vi "Write then Read.vi"(8 "error in (no error)":errorcluster, 9 "milliseconds to wait":u32, 10 "Write":string, 11 "Serial in":refnum<class "Serial.lvclass">) -> (0 "error out":errorcluster, 2 "Read":string, 3 "Serial out":refnum<class "Serial.lvclass">)   [LabVIEW 2021, in "Serial.lvclass"]
uses:
  Serial.lvclass
  Serial.lvclass/Serial.ctl
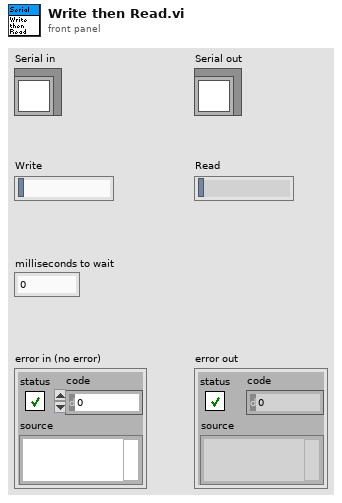
[diagram p1: front panel]
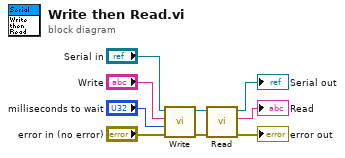
[diagram p0: block diagram]
diagram:
  n1 = call-dynamic "Write.vi"("error in (no error)"="error in (no error)", "milliseconds to wait"="milliseconds to wait", "Write"="Write", "Serial in"="Serial in") -> ("error out"=w4:errorcluster, "Serial out"=w8:refnum<class "Serial.lvclass">)  [unwired: 6 in]
  n2 = call-dynamic "Read.vi"("error in (no error)"=w4, "Serial in"=w8) -> ("error out"=→"error out":errorcluster, "Read"=→"Read":string, "Serial out"=→"Serial out":refnum<class "Serial.lvclass">)  [unwired: 7 in]
